vi "globalSetUp.vi"(8 "error in":errorcluster, 11 "Create Execution Unit in":refnum<class "Create Execution Unit.lvclass">) -> (0 "error out":errorcluster, 3 "Create Execution Unit out":refnum<class "Create Execution Unit.lvclass">)   [LabVIEW 2020, in "Create Execution Unit.lvclass"]
uses:
  Create Execution Unit.lvclass
  Hardware API/Global - Disable Hardware API Constant.vi
  Hardware API/AIM MIL-STD-1553 Hardware API.lvlib
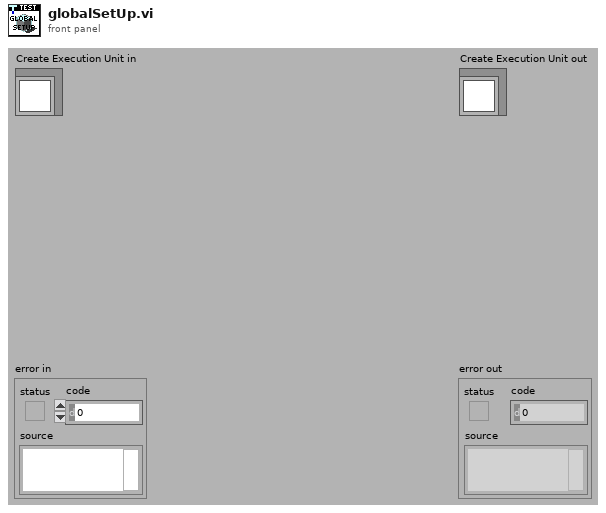
[diagram p1: front panel]
types:
  T1 = enum16{"Enabled (Default)", "Disabled for Unit Testing"}
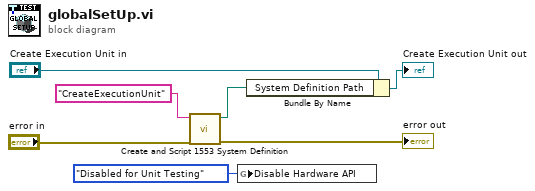
[diagram p0: block diagram]
diagram:
  n1 = call "Create and Script 1553 System Definition.vi"("error in"="error in", "System Definition Name"="CreateExecutionUnit") -> ("error out"=→"error out":errorcluster, "System Definition Path"=w6:path)  [unwired: 8 in]
  n2 = global write "Global - Disable Hardware API Constant.vi" "Disable Hardware API"(T1."Disabled for Unit Testing" ("Disable Hardware API")) -> ()
  n3 = Bundle By Name(cluster="Create Execution Unit in", "System Definition Path"=w6) -> (→"Create Execution Unit out":refnum<class "Create Execution Unit.lvclass">)
